vi "Arry_TO_DATA.vi"(9 "Param":T1={"Common"={"Velocity range"={"output high"=29.0, "output low"=-29.0}, "Vel_BasePos"=5, "Ref.Load_FindBase_L"=2.0, "Ref.Load_FindBase_R"=2.0, "Force_Peak"=150.0}, "Param_Left"={"L_기준값"=90.0, "L_검출값"=120.0, "L_End %"=42, "L_Onset %"=4, "L_Peak %"=28, "L_Pos"=0, "L_Offset"=0.0}, "Param_Right"={"R_기준값"=90.0, "R_검출값"=120.0, "R_End %"=42, "R_Onset %"=4, "R_Peak %"=28, "R_Pos"=0, "R_Offset"=0.0}}, 11 "DATA":sgl[][](array[numeric])) -> (0 "RIGHT":T2, 1 "LEFT":T2, 2 "IMU":sgl[][](array[numeric]), 3 "LoadCell":sgl[][](array[numeric]), 5 "PosVel":sgl[][](array[numeric]))   [LabVIEW 2023]
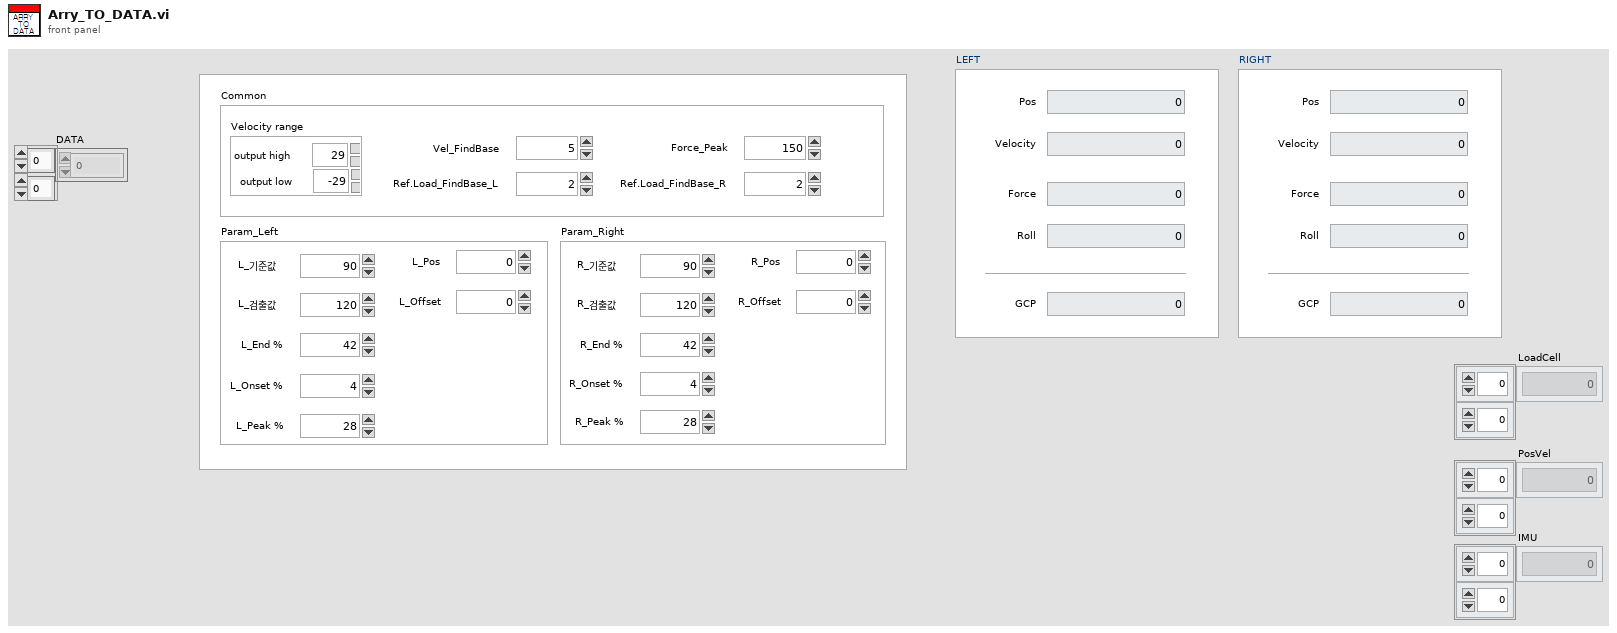
[diagram p1: front panel]
types:
  T1 = cluster{"Common":cluster{"Velocity range":cluster{"output high":dbl, "output low":dbl}, "Vel_BasePos":i32, "Ref.Load_FindBase_L":dbl, "Ref.Load_FindBase_R":dbl, "Force_Peak":dbl}, "Param_Left":cluster{"L_기준값":sgl, "L_검출값":sgl, "L_End %":i32, "L_Onset %":i32, "L_Peak %":i32, "L_Pos":i32, "L_Offset":sgl}, "Param_Right":cluster{"R_기준값":sgl, "R_검출값":sgl, "R_End %":i32, "R_Onset %":i32, "R_Peak %":i32, "R_Pos":i32, "R_Offset":sgl}}
  T2 = cluster{"Pos":sgl, "Velocity":sgl, "Force":sgl, "Roll":sgl, "GCP":sgl}
  T3 = cluster{"R_Pos":sgl, "R_Velocity":sgl, "R_Force":sgl, "R_Roll":sgl, "R_GCP":sgl}
  T4 = cluster{"L_Pos":sgl, "L_Velocity":sgl, "L_Force":sgl, "L_Roll":sgl, "L_GCP":sgl}
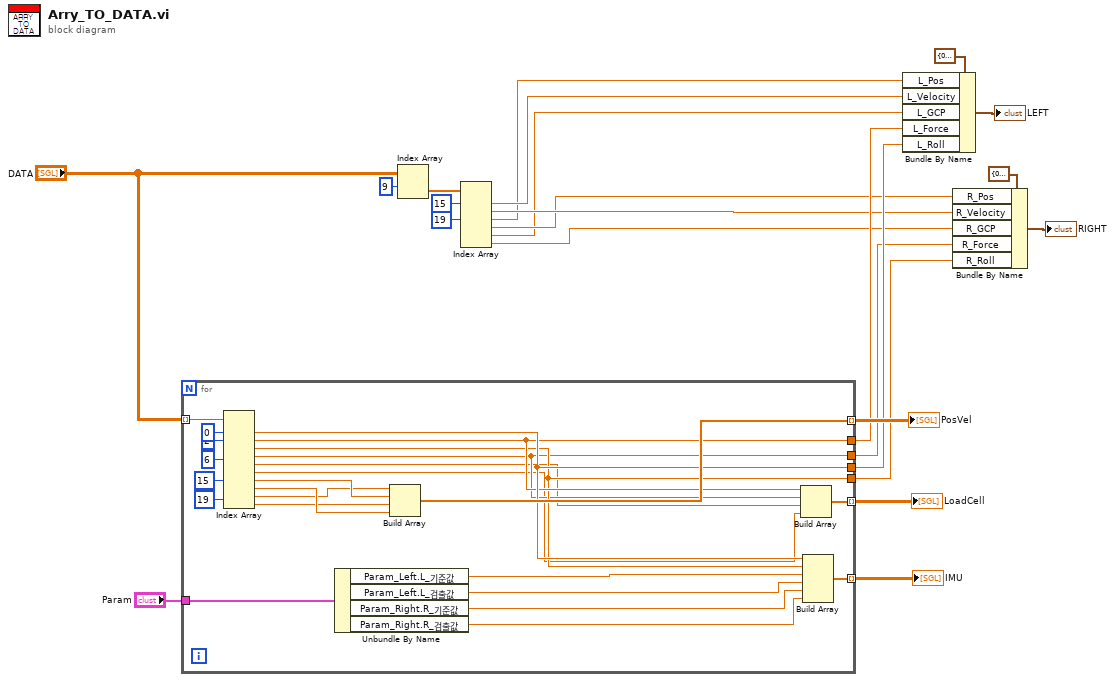
[diagram p0: block diagram]
diagram:
  n1 = for {
    tunnel: "DATA" -> [w39] mode=indexing
    tunnel: "Param" -> [w47]
    tunnel: [w42] -> w22 mode=indexing
    tunnel: [w35] -> w19
    tunnel: [w33] -> w15
    tunnel: [w37] -> w18
    tunnel: [w34] -> w14
    tunnel: [w41] -> w21 mode=indexing
    tunnel: [w40] -> w20 mode=indexing
    n2 = Index Array(array=w39, index #1=0 ("인덱스"), index #2=2 ("인덱스"), index #4=6 ("인덱스"), index #7=15 ("인덱스"), index #9=19 ("인덱스")) -> (element #1=w37:sgl, element #2=w35:sgl, element #3=w34:sgl, element #4=w33:sgl, element #5=w31:sgl, element #6=w30:sgl, element #7=w28:sgl, element #8=w27:sgl, element #9=w26:sgl, element #10=w25:sgl)  [unwired: 5 in]
    n3 = Unbundle By Name(w47) -> ("Param_Left.L_기준값"=w46:sgl, "Param_Left.L_검출값"=w45:sgl, "Param_Right.R_기준값"=w44:sgl, "Param_Right.R_검출값"=w43:sgl)
    n4 = Build Array(w26, w28, w25, w27) -> (w41:sgl[])
    n5 = Build Array(w35, w33, w31, w30) -> (w40:sgl[])
    n6 = Build Array(w37, w34, w46, w45, w44, w43) -> (w42:sgl[])
  }
  "LoadCell" <- w20
  "IMU" <- w22
  "PosVel" <- w21
  n7 = Index Array(array="DATA", index (row)=9 ("인덱스")) -> (element=w10:sgl[])  [unwired: 1 in]
  n8 = Index Array(array=w10, index #1=15 ("인덱스"), index #3=19 ("인덱스")) -> (element #1=w8:sgl, element #2=w7:sgl, element #3=w6:sgl, element #4=w5:sgl, element #5=w4:sgl, element #6=w3:sgl)  [unwired: 4 in]
  n9 = Bundle By Name(cluster=T4 {"L_Pos"=0.0, "L_Velocity"=0.0, "L_Force"=0.0, "L_Roll"=0.0, "L_GCP"=0.0} ("LEFT"), "L_Pos"=w6, "L_Velocity"=w8, "L_GCP"=w4, "L_Force"=w19, "L_Roll"=w18) -> (→"LEFT":T4)
  n10 = Bundle By Name(cluster=T3 {"R_Pos"=0.0, "R_Velocity"=0.0, "R_Force"=0.0, "R_Roll"=0.0, "R_GCP"=0.0} ("RIGHT"), "R_Pos"=w5, "R_Velocity"=w7, "R_GCP"=w3, "R_Force"=w15, "R_Roll"=w14) -> (→"RIGHT":T3)
